vi "MSScript_Format_Stop.vi"(11 "MSScript in":refnum<class "MSScript.lvclass">) -> (3 "Data":variant, 4 "#ofParamError":bool)   [LabVIEW 2018, in "MSScript.lvclass"]
uses:
  MSScript.lvclass
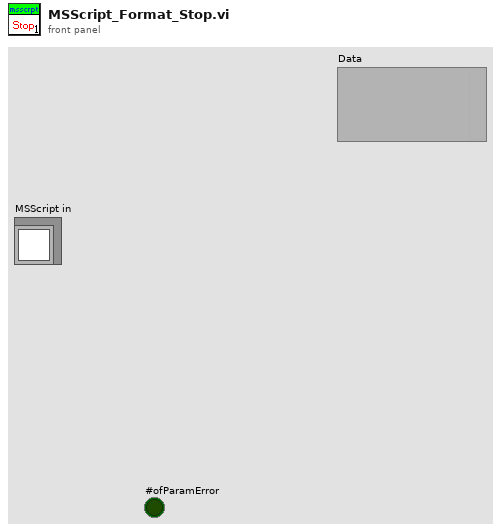
[diagram p1: front panel]
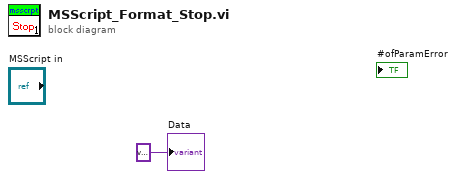
[diagram p0: block diagram]
diagram:
  "Data" <- variant
